vi "GetSavedSeq.vi"(7 "Reverse?":bool, 8 "error in (no error)":errorcluster, 9 "RF Points":u32, 10 "Channels to Acq":i32=1, 11 "instrument handle":refnum<k15>) -> (0 "error out":errorcluster, 1 "Samp Rate":sgl format="%.2e", 2 "Data":i16[][][](array[numeric]), 3 "instrument handle out":refnum<k15>, 5 "Att (dB)":dbl[](array[numeric]) format="%.2f")   [LabVIEW 2022 SP3]
uses:
  Motion Controllers/-MotionRoutines/MotionGlobals.vi
panel:
  in  "Case Constant\n(See Context Help)":bool
  out "Data Points":u32
  out "FS Volt pp":dbl format="%.2f"
  out "V/ div":string
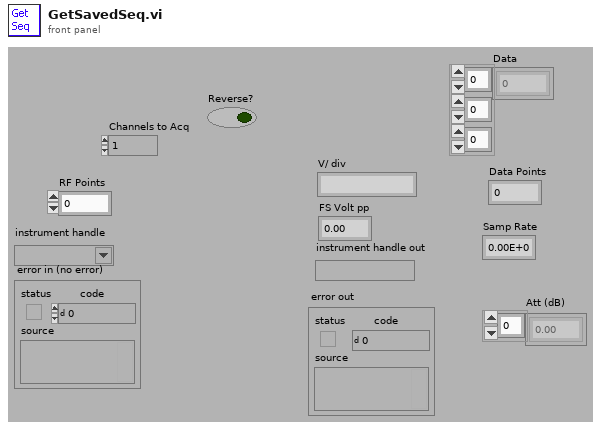
[diagram p1: front panel]
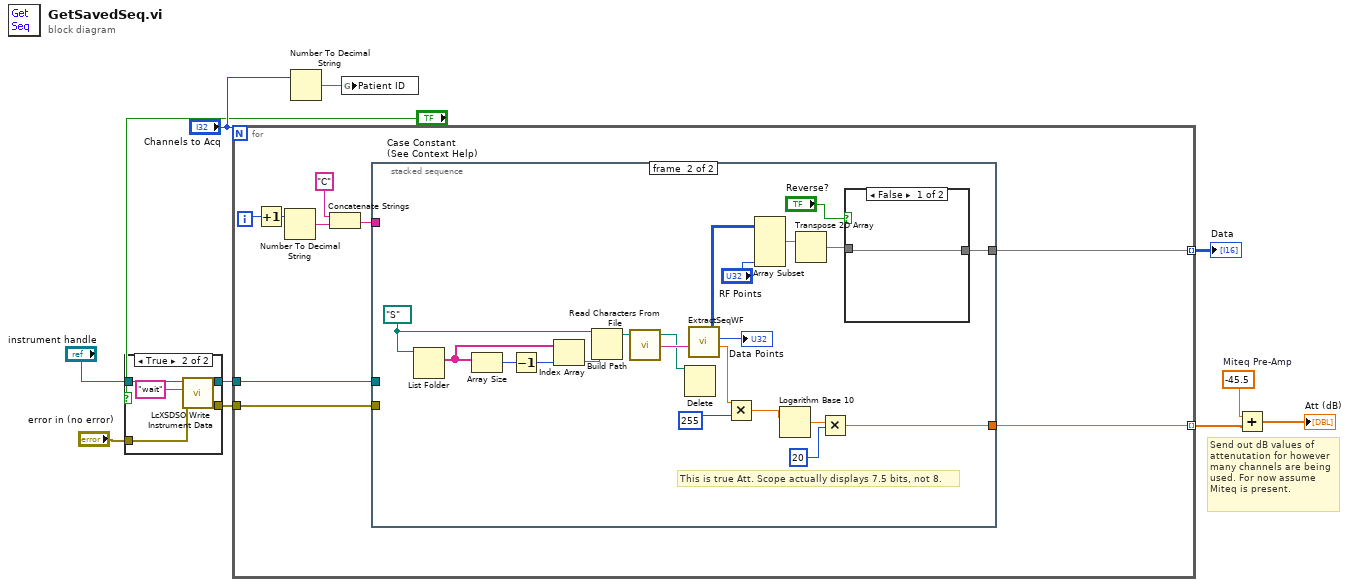
[diagram p0: block diagram]
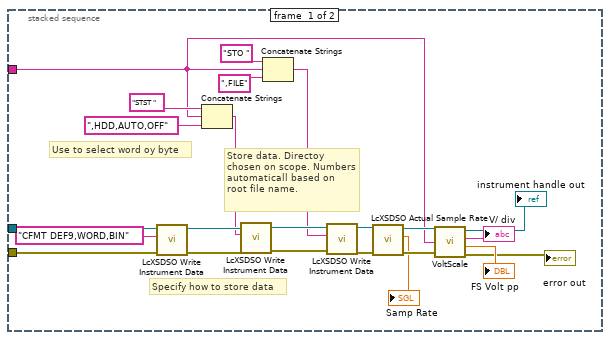
[diagram p3: hidden frame]
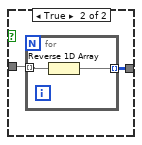
[diagram p4: hidden frame]
diagram:
  w6 = -45.5  # Miteq Pre-Amp
  # "Send out dB values of attenutation for however many channels are being used. For now assume Miteq is present."
  n1 = case shown="True" "Case Constant\n(See Context Help)" {
    tunnel: "instrument handle" -> [w13 w18]
    tunnel: [w13 w17] -> w4
    tunnel: [w12 w16] -> w3
    tunnel: "error in (no error)" -> [w12 w15]
    frame False {
    }
    frame True {
      n2 = call "LcXSDSO Write Instrument Data.vi"("error in (no error)"=w15, "write buffer"="wait", "instrument handle"=w18) -> ("error out"=w16:errorcluster, "instrument handle out"=w17:refnum<k15>)  [unwired: 7 in]
    }
  }
  n3 = for {
    N: "Channels to Acq" -> [_]
    tunnel: [w23] -> w11 mode=indexing
    tunnel: [w21] -> w8 mode=indexing
    tunnel: w4 -> [w20]
    tunnel: w3 -> [w19]
    i -> [w22]
    n4 = Increment(x=w22) -> (x+1=w24:i32)
    n5 = Number To Decimal String(number=w24) -> (decimal integer string=w25:string)  [unwired: 1 in]
    n6 = Concatenate Strings("C", w25) -> (w26:string)
    n7 = stacked-sequence {
      tunnel: w26 -> [w30 _]
      tunnel: [_ w53] -> w23
      tunnel: [_ w51] -> w21
      tunnel: w20 -> [w29 _]
      tunnel: w19 -> [w28 _]
      frame #0 {
        # "Store data. Directoy chosen on scope. Numbers automaticall based on root file name."
        # "Specify how to store data"
        # "Use to select word oy byte"
        n8 = call "LcXSDSO Write Instrument Data.vi"("error in (no error)"=w28, "write buffer"="CFMT DEF9,WORD,BIN", "instrument handle"=w29) -> ("error out"=w48:errorcluster, "instrument handle out"=w49:refnum<k15>)  [unwired: 7 in]
        n9 = Concatenate Strings("STST ", w30, ",HDD,AUTO,OFF") -> (w31:string)
        n10 = call "LcXSDSO Write Instrument Data.vi"("error in (no error)"=w48, "write buffer"=w31, "instrument handle"=w49) -> ("error out"=w46:errorcluster, "instrument handle out"=w47:refnum<k15>)  [unwired: 7 in]
        n11 = Concatenate Strings("STO ", w30, ",FILE") -> (w34:string)
        n12 = call "LcXSDSO Write Instrument Data.vi"("error in (no error)"=w46, "write buffer"=w34, "instrument handle"=w47) -> ("error out"=w40:errorcluster, "instrument handle out"=w41:refnum<k15>)  [unwired: 7 in]
        n13 = call "LcXSDSO Actual Sample Rate.vi"("error in (no error)"=w40, "instrument handle"=w41) -> ("error out"=w38:errorcluster, "sample rate"=→"Samp Rate":dbl, "instrument handle out"=w39:refnum<k15>)  [unwired: 7 in]
        n14 = call "VoltScale.vi"("instrument handle in"=w39, "Channel name"=w30, "error in"=w38) -> ("inst handle OUT"=→"instrument handle out":refnum<k15>, "V/ div"=→"V/ div":string, "FS Volt pp"=→"FS Volt pp":dbl, "error out"=→"error out":errorcluster)  [unwired: 1 in]
      }
      frame #1 {
        w66 = path "S:/" ("file path (dialog if empty)")
        # "This is true Att. Scope actually displays 7.5 bits, not 8."
        n15 = List Folder(path=w66) -> (filenames=w67:string[])  [unwired: 3 in, 3 out]
        n16 = Array Size(array=w67) -> (size(s)=w69:i32)
        n17 = Decrement(x=w69) -> (x-1=w68:i32)
        n18 = Index Array(array=w67, index=w68) -> (element=w65:string)
        n19 = Build Path(base path=w66, name or relative path=w65) -> (appended path=w64:path)
        n20 = call <vilib>:"Read Characters From File.vi"("file path (dialog if empty)"=w64) -> ("new file path (NotAPath if cancelled)"=w63:path, "character string"=w71:string)  [unwired: 5 in, 2 out]
        n21 = Delete(path (use dialog)=w63) -> ()  [unwired: 4 in, 3 out]
        n22 = call "ExtractSeqWF.vi"("String"=w71) -> ("vert gain"=w60:sgl, "Data Pts"=→"Data Points":i32, "Data"=w56:i8[][])  [unwired: 4 in]
        n23 = Multiply(x=w60, y=255) -> (x*y=w58:sgl)
        n24 = Array Subset(array=w56, length (col)="RF Points") -> (w55:i8[][])  [unwired: 3 in]
        n25 = Logarithm Base 10(1:w58) -> (0:w61:sgl)
        n26 = Transpose 2D Array(2D array=w55) -> (transposed array=w54:i8[][])
        n27 = Multiply(x=w61, y=20) -> (x*y=w51:sgl)
        n28 = case shown="False" "Reverse?" {
          tunnel: w54 -> [w72 w73]
          tunnel: [w72 w74] -> w53
          frame False {
          }
          frame True {
            n29 = for {
              tunnel: w73 -> [w76] mode=indexing
              tunnel: [w75] -> w74 mode=indexing
              n30 = Reverse 1D Array(array=w76) -> (reversed array=w75:i8[])
            }
          }
        }
      }
    }
  }
  "Data" <- w11
  n31 = Number To Decimal String(number="Channels to Acq") -> (decimal integer string=w9:string)  [unwired: 1 in]
  n32 = global write "MotionGlobals.vi" "Patient ID"(w9) -> ()
  n33 = Add(x=w6, y=w8) -> (x+y=→"Att (dB)":dbl[])
